vi "CSMOMgr-Create CSMO.vi"(7 "Allowed Messages (Empty For All)":string[](array[string]), 8 "error in (no error)":errorcluster, 10 "Name (\"\" to Use UUID) In":string, 11 "CSMOMgr":T1) -> (0 "error out":errorcluster, 2 "CSMO":T2, 3 "CSMOMgr Out":T1)   [LabVIEW 2017, in "Communicable State Machine.lvlib"]
uses:
  Communicable State Machine.lvlib
  Def-CSMOMgr.ctl
  CSMQ/_CSMObj.ctl
  CSMQ/_CSMObj-Info.ctl
  Typedef/_CSM_MODE.ctl
  CSMQ/_CSMObj-Refs.ctl
  CSMQ/_CSMObj-Data.ctl
  Priority Queue/Priority Queue.ctl
  Typedef/_Cross CSM State Data.ctl
  Typedef/_CSM_MSG_TYPE.ctl
  Typedef/_Cross CSM State Response.ctl
  Typedef/_CSM_Response Source Message.ctl
  Priority Queue/def-Data(LowPRI-Q).ctl
  CSMQ/_CSMObj-ModeData.ctl
  Typedef/_CSM Status Change Event Data.ctl
  Error/CSM Invalid Name Error.vi
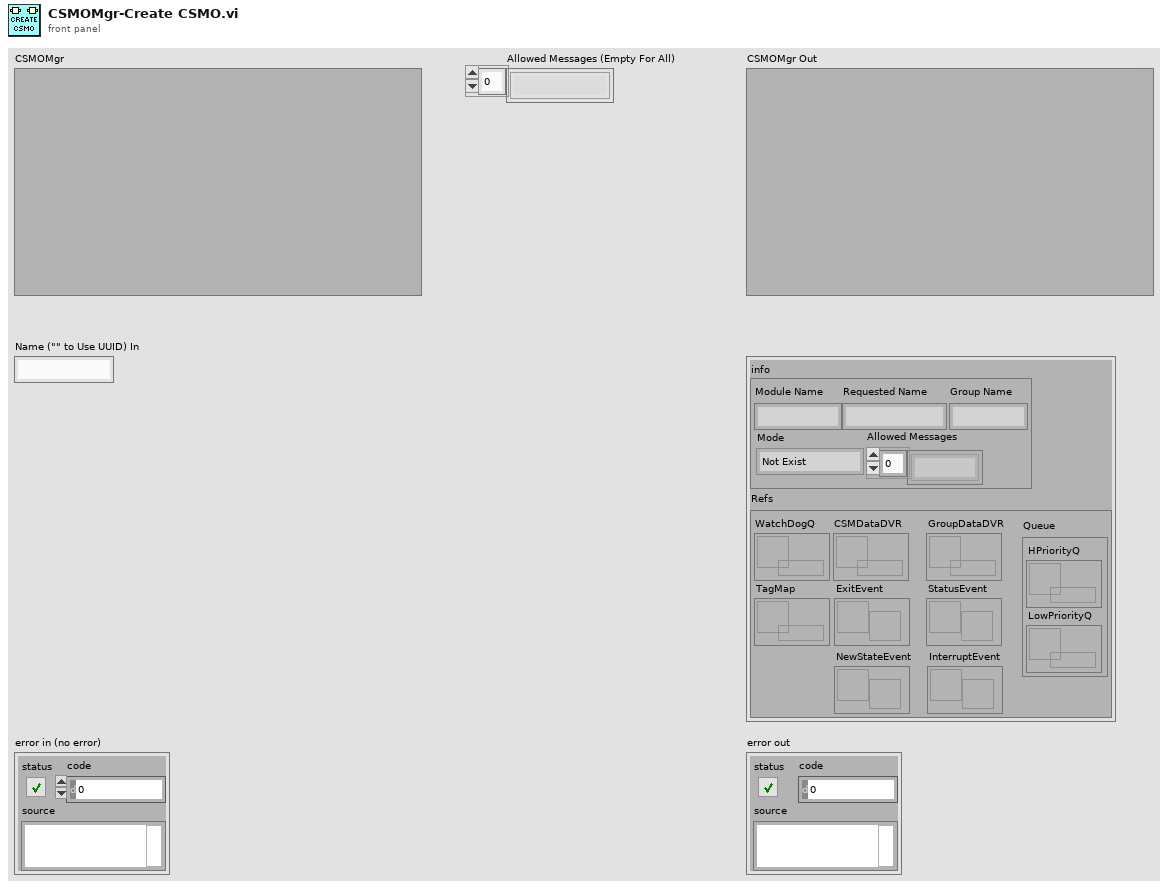
[diagram p1: front panel]
types:
  T1 = typedef "Communicable State Machine.lvlib/Def-CSMOMgr.ctl" = variant
  T2 = typedef "Communicable State Machine.lvlib/_CSMObj.ctl" = cluster{"info":T3, "Refs":T5}
  T3 = typedef "Communicable State Machine.lvlib/_CSMObj-Info.ctl" = cluster{"Module Name":string, "Requested Name":string, "Group Name":string, "Mode":T4, "Allowed Messages":string[]}
  T4 = typedef "Communicable State Machine.lvlib/_CSM_MODE.ctl" = enum16{"Not Exist", "Stand Alone", "CSM", "Worker", "Worker Agent", "Chain Node", "Chain"}
  T5 = typedef "Communicable State Machine.lvlib/_CSMObj-Refs.ctl" = cluster{"WatchDogQ":refnum<queue>, "CSMDataDVR":refnum<data-value>, "Queue":T6, "GroupDataDVR":refnum<data-value>, "TagMap":refnum<data-value>, "ExitEvent":refnum<user-event>, "NewStateEvent":refnum<user-event>, "StatusEvent":refnum<user-event>, "InterruptEvent":refnum<user-event>}
  T6 = typedef "Communicable State Machine.lvlib/Priority Queue.ctl" = cluster{"HPriorityQ":refnum<queue>, "LowPriorityQ":refnum<queue>}
  T7 = typedef "Communicable State Machine.lvlib/_CSM_NAME_REQUEST.ctl" = enum16{"Stand Alone CSM Request", "Normal CSM Request", "Agent Request", "Action Worker Request", "Chain Request", "Chain Node Request"}
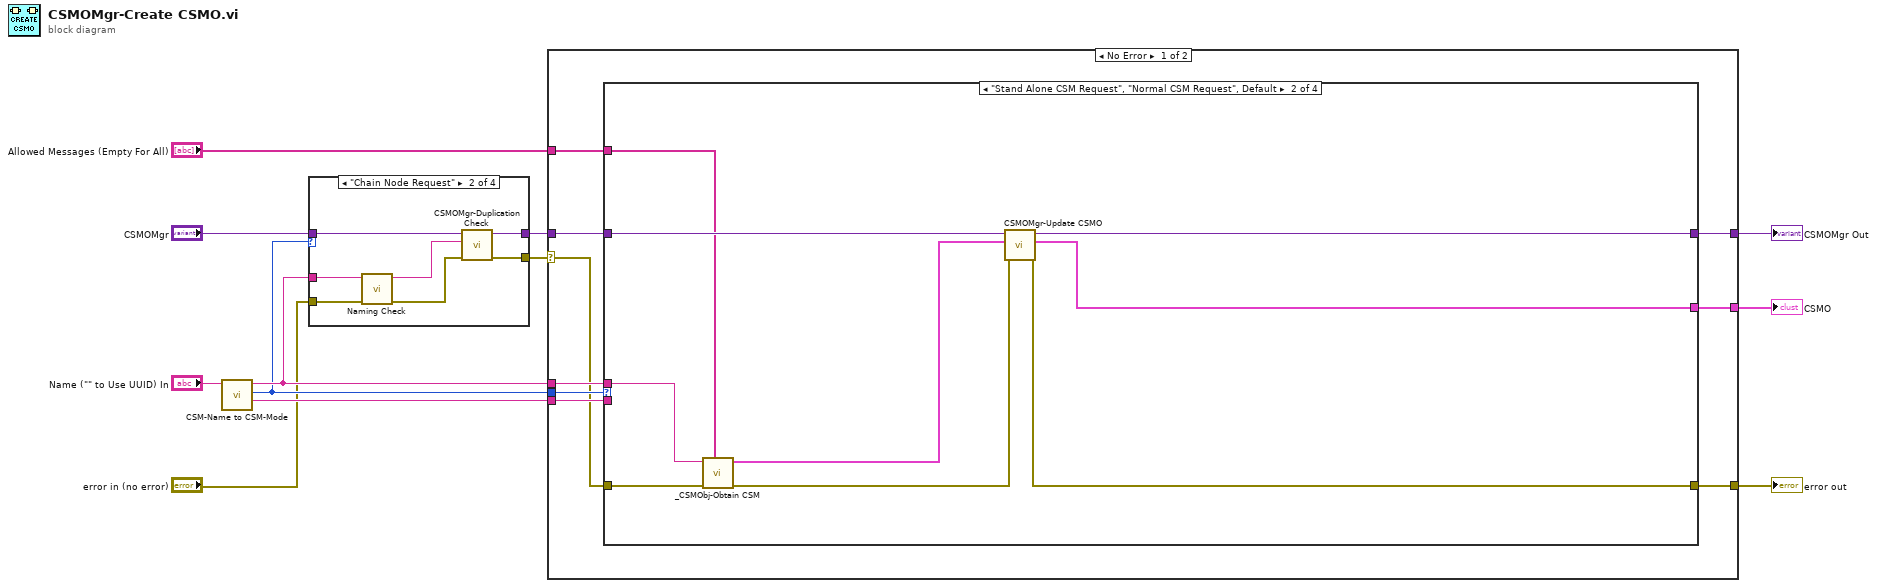
[diagram p0: block diagram]
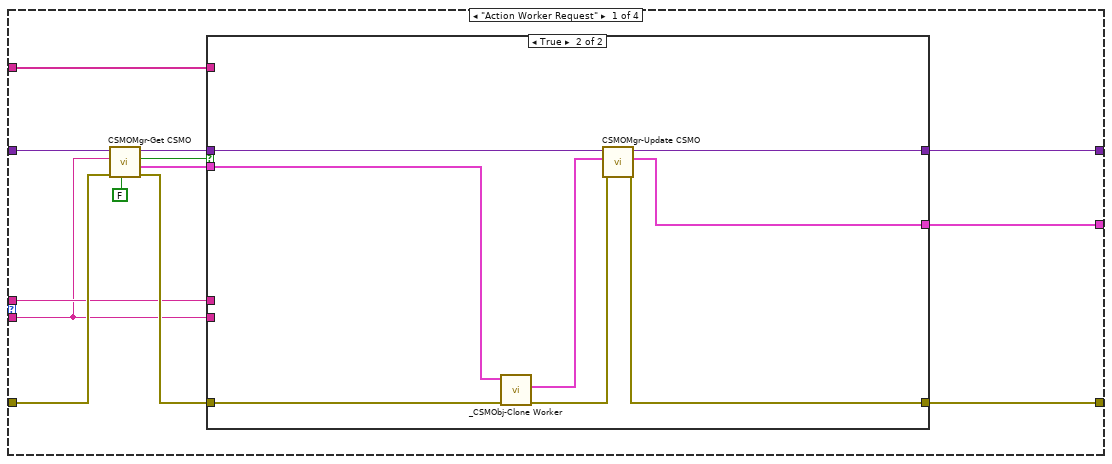
[diagram p2: hidden frame]
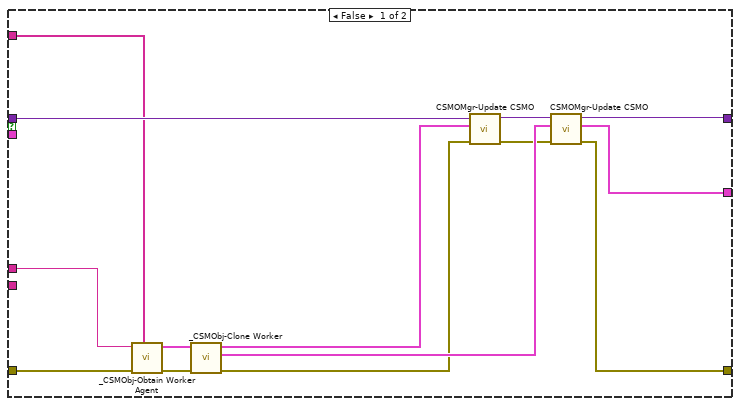
[diagram p3: hidden frame]
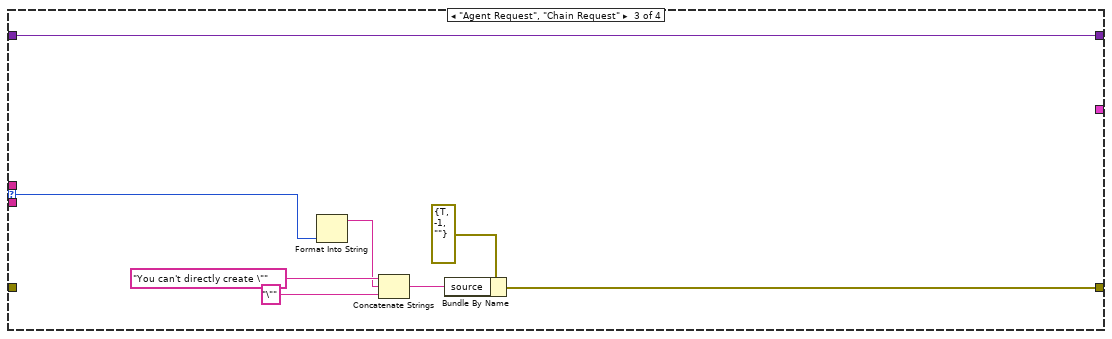
[diagram p4: hidden frame]
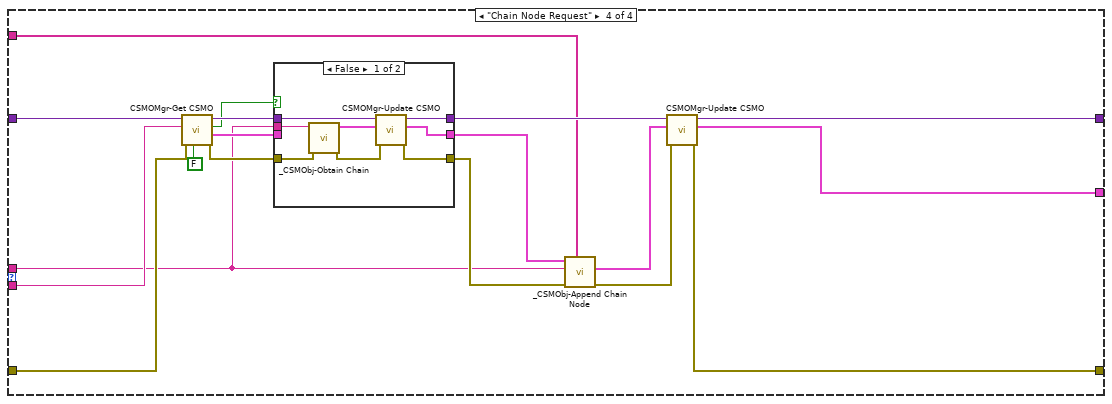
[diagram p5: hidden frame]
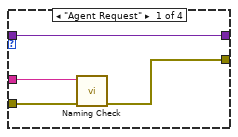
[diagram p8: hidden frame]
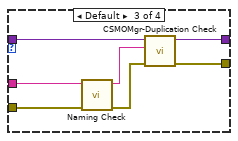
[diagram p9: hidden frame]
diagram:
  n1 = call "CSM-Name to CSM-Mode.vi"("String"="Name (\"\" to Use UUID) In") -> ("ParentCSM Name"=w10:string, "CSM Mode"=w11:T7, "Requested Name"=w12:string)  [unwired: 8 in]
  n2 = case shown="\"Chain Node Request\"" w11 {
    tunnel: [w14 w20 w30 w32] -> w6
    tunnel: [w13 w18 w28 w31] -> w7
    tunnel: "CSMOMgr" -> [w14 w21 w26 w32]
    tunnel: "error in (no error)" -> [w15 w22 w25 w31]
    tunnel: w12 -> [w16 w23 w24 _]
    frame "Agent Request" {
      n3 = call "Naming Check.vi"("error in (no error)"=w15, "Name (\"\" to Use UUID)"=w16) -> ("error out"=w13:errorcluster)  [unwired: 8 in, 1 out]
    }
    frame "Chain Node Request" {
      n4 = call "Naming Check.vi"("error in (no error)"=w22, "Name (\"\" to Use UUID)"=w23) -> ("error out"=w17:errorcluster, "Name (Dup)"=w19:string)  [unwired: 8 in]
      n5 = call "CSMOMgr-Duplication Check.vi"("Error In"=w17, "Queue Name"=w19, "CSMOMgr"=w21) -> ("error out"=w18:errorcluster, "CSMOMgr Out"=w20:T1)  [unwired: 7 in]
    }
    frame Default {
      n6 = call "Naming Check.vi"("error in (no error)"=w25, "Name (\"\" to Use UUID)"=w24) -> ("error out"=w29:errorcluster, "Name (Dup)"=w27:string)  [unwired: 8 in]
      n7 = call "CSMOMgr-Duplication Check.vi"("Error In"=w29, "Queue Name"=w27, "CSMOMgr"=w26) -> ("error out"=w28:errorcluster, "CSMOMgr Out"=w30:T1)  [unwired: 7 in]
    }
    frame "Stand Alone CSM Request" {
    }
  }
  n8 = case shown="No Error" w7 {
    selector: w7 -> [w38 w124]
    tunnel: w12 -> [w41 _]
    tunnel: w11 -> [w40 _]
    tunnel: w10 -> [w39 _]
    tunnel: w6 -> [w37 w123]
    tunnel: "Allowed Messages (Empty For All)" -> [w36 _]
    tunnel: [w35 w124] -> w3
    tunnel: [w34 w123] -> w2
    tunnel: [w33 _] -> w1
    frame No Error {
      n9 = case shown="\"Stand Alone CSM Request\", \"Normal CSM Request\", Default" w40 {
        selector: w40 -> [_ _ w87 _]
        tunnel: [w54 w85 w93 w101] -> w34
        tunnel: [w53 w84 w89 w97] -> w35
        tunnel: w36 -> [w52 w78 _ w96]
        tunnel: [w51 w81 _ w99] -> w33
        tunnel: w37 -> [w47 w83 w93 w110]
        tunnel: w38 -> [w46 w82 _ w109]
        tunnel: w41 -> [w43 w77 _ w94]
        tunnel: w39 -> [w42 _ _ w108]
        frame "Action Worker Request" {
          n10 = call "CSMOMgr-Get CSMO.vi"("GenError? (T)"=FALSE ("GenError?(T)"), "Error In"=w46, "Queue Name"=w42, "CSMOMgr"=w47) -> ("error out"=w48:errorcluster, "Values"=w49:T2, "Found"=w45:bool, "CSMOMgr Out"=w50:T1)  [unwired: 4 in]
          n11 = case shown="True" w45 {
            tunnel: [w58 w69] -> w51
            tunnel: w50 -> [w68 w73]
            tunnel: [w64 w72] -> w54
            tunnel: w49 -> [_ w76]
            tunnel: w48 -> [w67 w75]
            tunnel: [w59 w70] -> w53
            tunnel: w43 -> [w55 _]
            tunnel: w52 -> [w66 _]
            tunnel: w42 -> [_ _]
            frame False {
              n12 = call "_CSMObj-Obtain Worker Agent.vi"("Allowed Messages (Empty For All)"=w66, "error in (no error)"=w67, "Requested Name"=w55) -> ("error out"=w56:errorcluster, "CSMQ Out"=w57:T2)  [unwired: 7 in]
              n13 = call "_CSMObj-Clone Worker.vi"("Error In"=w56, "CSMObj In"=w57) -> ("error out"=w61:errorcluster, "Output Cluster"=w63:T2, "CSMObj Out"=w62:T2)  [unwired: 7 in]
              n14 = call "CSMOMgr-Update CSMO.vi"("error in (no error)"=w61, "CSMO"=w62, "CSMOMgr In"=w68) -> ("error out"=w60:errorcluster, "CSMOMgr Out"=w65:T1)  [unwired: 6 in, 1 out]
              n15 = call "CSMOMgr-Update CSMO.vi"("error in (no error)"=w60, "CSMO"=w63, "CSMOMgr In"=w65) -> ("error out"=w59:errorcluster, "CSMO (Dup)"=w58:T2, "CSMOMgr Out"=w64:T1)  [unwired: 6 in]
            }
            frame True {
              n16 = call "_CSMObj-Clone Worker.vi"("Error In"=w75, "CSMObj In"=w76) -> ("error out"=w71:errorcluster, "Output Cluster"=w74:T2)  [unwired: 7 in, 1 out]
              n17 = call "CSMOMgr-Update CSMO.vi"("error in (no error)"=w71, "CSMO"=w74, "CSMOMgr In"=w73) -> ("error out"=w70:errorcluster, "CSMO (Dup)"=w69:T2, "CSMOMgr Out"=w72:T1)  [unwired: 6 in]
            }
          }
        }
        frame "Stand Alone CSM Request", "Normal CSM Request", Default {
          n18 = call "_CSMObj-Obtain CSM.vi"("Allowed Messages (Empty For All)"=w78, "error in (no error)"=w82, "Requested Name"=w77) -> ("error out"=w79:errorcluster, "CSMQ Out"=w80:T2)  [unwired: 7 in]
          n19 = call "CSMOMgr-Update CSMO.vi"("error in (no error)"=w79, "CSMO"=w80, "CSMOMgr In"=w83) -> ("error out"=w84:errorcluster, "CSMO (Dup)"=w81:T2, "CSMOMgr Out"=w85:T1)  [unwired: 6 in]
        }
        frame "Agent Request", "Chain Request" {
          n20 = Format Into String(w87) -> (resulting string=w86:string)  [unwired: 3 in, 1 out]
          n21 = Concatenate Strings("You can't directly create \"" ("source"), w86, "\"" ("source")) -> (w88:string)
          n22 = Bundle By Name(cluster=errorcluster {"status"=TRUE, "code"=-1, "source"=""} ("error out"), "source"=w88) -> (w89:errorcluster)
        }
        frame "Chain Node Request" {
          n23 = call "CSMOMgr-Get CSMO.vi"("GenError? (T)"=FALSE ("GenError?(T)"), "Error In"=w109, "Queue Name"=w108, "CSMOMgr"=w110) -> ("error out"=w107:errorcluster, "Values"=w105:T2, "Found"=w104:bool, "CSMOMgr Out"=w106:T1)  [unwired: 4 in]
          n24 = case shown="False" w104 {
            tunnel: w94 -> [w119 _]
            tunnel: w107 -> [w118 w121]
            tunnel: [w117 w121] -> w95
            tunnel: w106 -> [w116 w120]
            tunnel: w105 -> [_ w122]
            tunnel: [w113 w122] -> w103
            tunnel: [w112 w120] -> w102
            frame False {
              n25 = call "_CSMObj-Obtain Chain.vi"("error in (no error)"=w118, "Requested Name"=w119) -> ("error out"=w115:errorcluster, "CSMQ Out"=w114:T2)  [unwired: 8 in]
              n26 = call "CSMOMgr-Update CSMO.vi"("error in (no error)"=w115, "CSMO"=w114, "CSMOMgr In"=w116) -> ("error out"=w117:errorcluster, "CSMO (Dup)"=w113:T2, "CSMOMgr Out"=w112:T1)  [unwired: 6 in]
            }
            frame True {
            }
          }
          n27 = call "_CSMObj-Append Chain Node.vi"("Allowed Messages (Empty For All)"=w96, "Error In"=w95, "Requested Name"=w94, "CSMObj In"=w103) -> ("error out"=w98:errorcluster, "Output Cluster (Dup)"=w100:T2)  [unwired: 5 in, 1 out]
          n28 = call "CSMOMgr-Update CSMO.vi"("error in (no error)"=w98, "CSMO"=w100, "CSMOMgr In"=w102) -> ("error out"=w97:errorcluster, "CSMO (Dup)"=w99:T2, "CSMOMgr Out"=w101:T1)  [unwired: 6 in]
        }
      }
    }
    frame Error {
    }
  }
  "CSMO" <- w1
  "error out" <- w3
  "CSMOMgr Out" <- w2
